vi "Y Axis Speed Conversion sub_VI.vi"(10 "Microsteps per Rev":T1(ring), 11 "Setpoint\nSpeed (mm/s)":dbl) -> (3 "PWM Frequency":dbl)   [LabVIEW 2017]
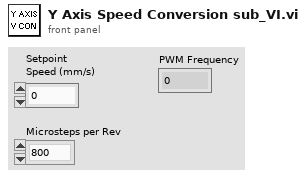
[diagram p1: front panel]
types:
  T1 = enum16{"800", "1600", "3200", "6400", "12800", "25600"}
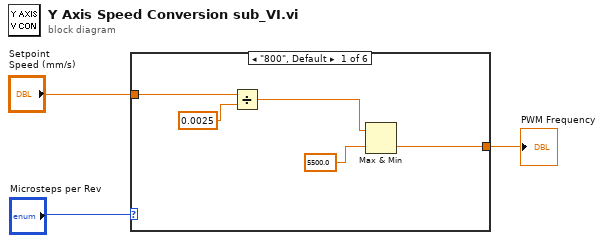
[diagram p0: block diagram]
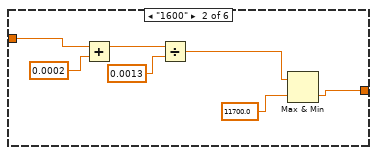
[diagram p2: hidden frame]
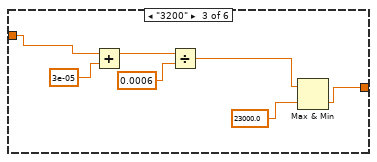
[diagram p3: hidden frame]
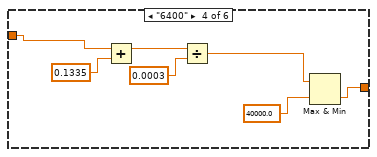
[diagram p4: hidden frame]
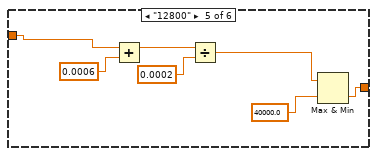
[diagram p5: hidden frame]
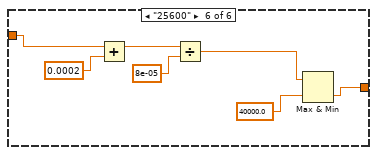
[diagram p6: hidden frame]
diagram:
  n1 = case shown="\"800\", Default" "Microsteps per Rev" {
    tunnel: "Setpoint\nSpeed (mm/s)" -> [w7 w11 w17 w24 w30 w38]
    tunnel: [w4 w12 w16 w23 w31 w37] -> w3
    frame "800", Default {
      n2 = Divide(x=w7, y=0.0025) -> (x/y=w6:dbl)
      n3 = Max & Min(x=w6, y=5500.0) -> (min(x,y)=w4:dbl)  [unwired: 1 out]
    }
    frame "1600" {
      n4 = Add(x=w11, y=0.0002) -> (x+y=w10:dbl)
      n5 = Divide(x=w10, y=0.0013) -> (x/y=w15:dbl)
      n6 = Max & Min(x=w15, y=11700.0) -> (min(x,y)=w12:dbl)  [unwired: 1 out]
    }
    frame "3200" {
      n7 = Add(x=w17, y=3e-05) -> (x+y=w19:dbl)
      n8 = Divide(x=w19, y=0.0006) -> (x/y=w22:dbl)
      n9 = Max & Min(x=w22, y=23000.0) -> (min(x,y)=w16:dbl)  [unwired: 1 out]
    }
    frame "6400" {
      n10 = Add(x=w24, y=0.1335) -> (x+y=w29:dbl)
      n11 = Divide(x=w29, y=0.0003) -> (x/y=w28:dbl)
      n12 = Max & Min(x=w28, y=40000.0) -> (min(x,y)=w23:dbl)  [unwired: 1 out]
    }
    frame "12800" {
      n13 = Add(x=w30, y=0.0006) -> (x+y=w35:dbl)
      n14 = Divide(x=w35, y=0.0002) -> (x/y=w36:dbl)
      n15 = Max & Min(x=w36, y=40000.0) -> (min(x,y)=w31:dbl)  [unwired: 1 out]
    }
    frame "25600" {
      n16 = Add(x=w38, y=0.0002) -> (x+y=w43:dbl)
      n17 = Divide(x=w43, y=8e-05) -> (x/y=w42:dbl)
      n18 = Max & Min(x=w42, y=40000.0) -> (min(x,y)=w37:dbl)  [unwired: 1 out]
    }
  }
  "PWM Frequency" <- w3
